vi "Wait For Operation Complete.vi"(8 "error in (no error)":errorcluster, 10 "Timeout [ms] (30000)":u32=30000, 11 "VISA resource name":refnum<visa-resource-name>) -> (0 "error out":errorcluster, 3 "VISA resource name out":refnum<visa-resource-name>)   [LabVIEW 2012, in "Tektronix TTR500 Series.lvlib"]
doc: "Waits for the operation to complete."
uses:
  <instrlib>/Tektronix TTR500 Series/Tektronix TTR500 Series.lvlib
panel:
  out "read buffer":string
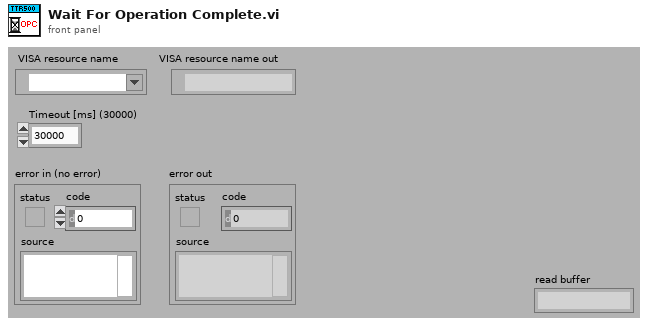
[diagram p1: front panel]
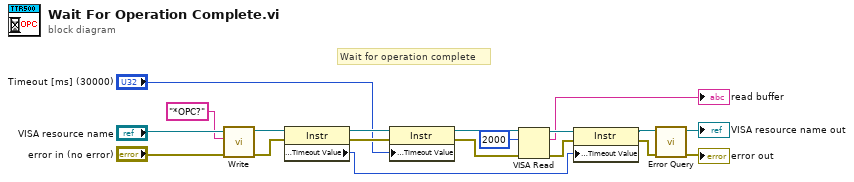
[diagram p0: block diagram]
diagram:
  # "Wait for operation complete"
  n1 = call <instrlib>:"Write.vi"("error in (no error)"="error in (no error)", "String ()"="*OPC?" ("write buffer"), "VISA resource name"="VISA resource name") -> ("error out"=w4:errorcluster, "VISA resource name out"=w5:refnum<visa-resource-name>)  [unwired: 6 in, 1 out]
  n2 = property class="Instr"(reference=w5, error in=w4) -> (reference out=w11:refnum<visa-resource-name>, error out=w10:errorcluster, "General Settings:Timeout Value"=w7:u32)
  n3 = property class="Instr"(reference=w11, error in=w10, "General Settings:Timeout Value"="Timeout [ms] (30000)") -> (reference out=w14:refnum<visa-resource-name>, error out=w13:errorcluster)
  n4 = VISA Read(VISA resource name=w14, byte count=u32 2000, error in (no error)=w13) -> (VISA resource name out=w9:refnum<visa-resource-name>, read buffer=→"read buffer":string, error out=w8:errorcluster)  [unwired: 1 out]
  n5 = property class="Instr"(reference=w9, error in=w8, "General Settings:Timeout Value"=w7) -> (reference out=w1:refnum<visa-resource-name>, error out=w2:errorcluster)
  n6 = call <instrlib>:"Error Query.vi"("error in (no error)"=w2, "VISA resource name"=w1) -> ("error out"=→"error out":errorcluster, "VISA resource name out"=→"VISA resource name out":refnum<visa-resource-name>)  [unwired: 6 in, 2 out]
